vi "getErrorInfo.vi"(8 "error in (no error)":errorcluster) -> (0 "error out":errorcluster, 3 "IErrorInfo out":refnum<class "IErrorInfo.lvclass">)   [LabVIEW 2022 SP3, in "openDAQ.lvlib" / "IBaseObject.lvlib" / "IErrorInfo.lvlib" / "IErrorInfo.lvclass"]
uses:
  <instrlib>/openDAQ/Public/Classes/IErrorInfo/IErrorInfo.lvclass
  C:/Program Files (x86)/National Instruments/LabVIEW 2022/instr.lib/openDAQ/Public/Classes/IBaseObject/IBaseObject.lvclass
  <instrlib>/openDAQ/Public/Classes/IBaseObject/IBaseObject.lvclass/IBaseObject.ctl
  <instrlib>/openDAQ/Public/Classes/IBaseObject/Accessor/Write reference.vi
  <instrlib>/openDAQ/Public/Classes/IErrorInfo/IErrorInfo.lvclass/IErrorInfo.ctl
  <instrlib>/openDAQ/Binaries/Windows/x86/daqcoretypes-32-3.dll
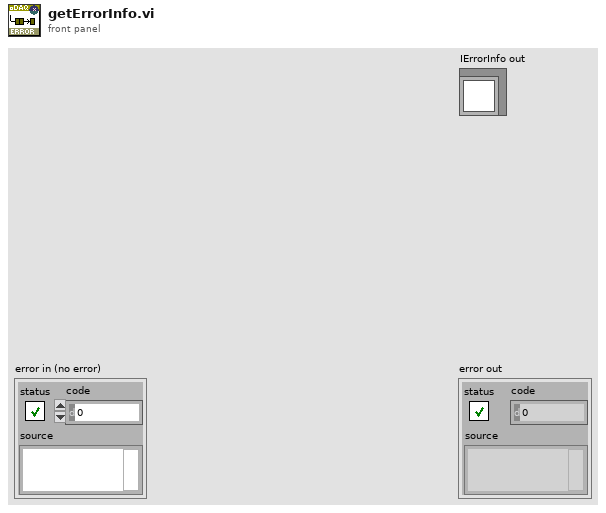
[diagram p1: front panel]
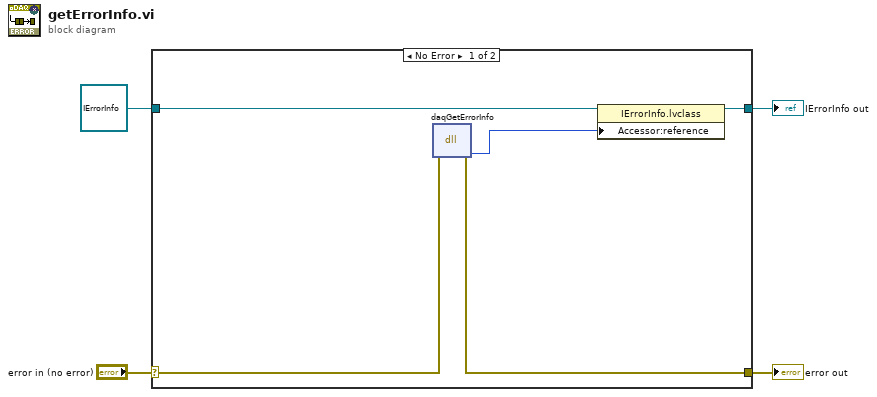
[diagram p0: block diagram]
diagram:
  n1 = case shown="No Error" "error in (no error)" {
    selector: "error in (no error)" -> [w8 w11]
    tunnel: [w7 w11] -> w3
    tunnel: [w6 w10] -> w1
    tunnel: refnum<class "IErrorInfo.lvclass"> refnum ("IErrorInfo in") -> [w9 w10]
    frame No Error {
      n2 = dll-call lib="C:/Program Files (x86)/National Instruments/LabVIEW 2022/instr.lib/openDAQ/Binaries/Windows/x86/daqcoretypes-*-3.*" fn="daqGetErrorInfo"(error in=w8) -> (error out=w7:errorcluster, "errorInfo"=w5:i64)  [unwired: 4 in, 1 out]
      n3 = property class="IErrorInfo.lvclass"(reference=w9, "Accessor:reference"=w5) -> (reference out=w6:refnum<class "IErrorInfo.lvclass">)  [unwired: 1 in, 1 out]
    }
    frame Error {
    }
  }
  "error out" <- w3
  "IErrorInfo out" <- w1
